vi "ModifyDefectDescription.vi"(2 "Bad Channel array":i32[](array[numeric]), 3 "Defect flag array":i32[](array[numeric]), 4 "Defect Number":i32) -> (0 "Defect flag array out":i32[](array[numeric]), 1 "Updated?":bool)   [LabVIEW 2018]
panel:
  out "Channel":i32
  out "is declared to be a":string
  in  "stop copy":bool
  in  "stop":bool
  in  "Change to:":u16(ring) items=["Pinhole", "Oxide-Punchthrough", "Short", "Open", "Resistor-Break", "Implant-Open", "Compliance exceeded"]
  # "Modify Strip Defect Description"
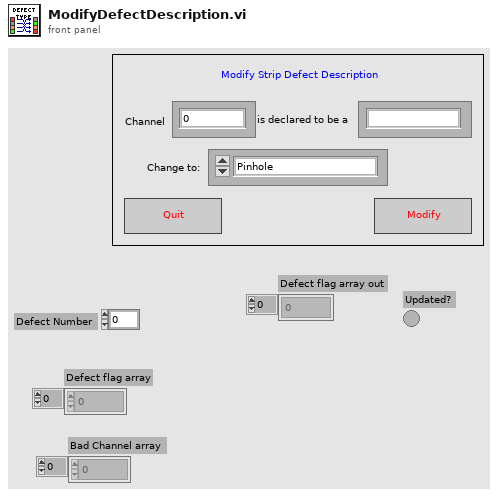
[diagram p1: front panel]
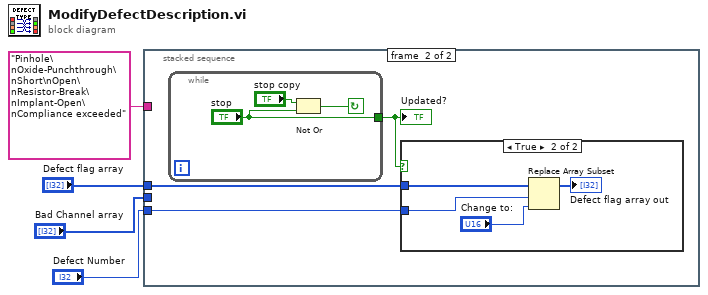
[diagram p0: block diagram]
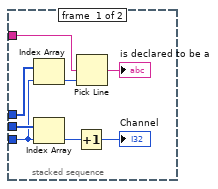
[diagram p2: hidden frame]
diagram:
  n1 = stacked-sequence {
    tunnel: "Bad Channel array" -> [w8 _]
    tunnel: "Defect Number" -> [w7 w14]
    tunnel: "Pinhole\nOxide-Punchthrough\nShort\nOpen\nResistor-Break\nImplant-Open\nCompliance exceeded" -> [w12 _]
    tunnel: "Defect flag array" -> [w9 w15]
    frame #0 {
      n2 = Index Array(array=w9, index=w7) -> (element=w11:i32)
      n3 = Index Array(array=w8, index=w7) -> (element=w5:i32)
      n4 = Increment(x=w5) -> (x+1=→"Channel":i32)
      n5 = Pick Line(multi-line string=w12, line index=w11) -> (output string=→"is declared to be a":string)  [unwired: 1 in]
    }
    frame #1 {
      n6 = while {
        tunnel: ["stop"] -> w13
        stop <- w22 continue-if-true
        n7 = Not Or(1:"stop", 2:"stop copy") -> (0:w22:bool)
      }
      "Updated?" <- w13
      n8 = case shown="True" w13 {
        tunnel: w15 -> [_ w19]
        tunnel: w14 -> [_ w17]
        frame False {
        }
        frame True {
          n9 = Replace Array Subset(array=w19, new element="Change to:", index=w17) -> (→"Defect flag array out":i32[])
        }
      }
    }
  }
